vi "Base Set Run Java Script Error.vi"(4 "error in":errorcluster, 5 "output file in":path, 6 "data in":T1, 7 "ATS Framework Fields in":T2) -> (0 "error out":errorcluster)   [LabVIEW 2019]
uses:
  ATS Framework Fields.ctl
  Run Tool Output.ctl
  <vilib>/regexp/Match Regular Expression.xnode
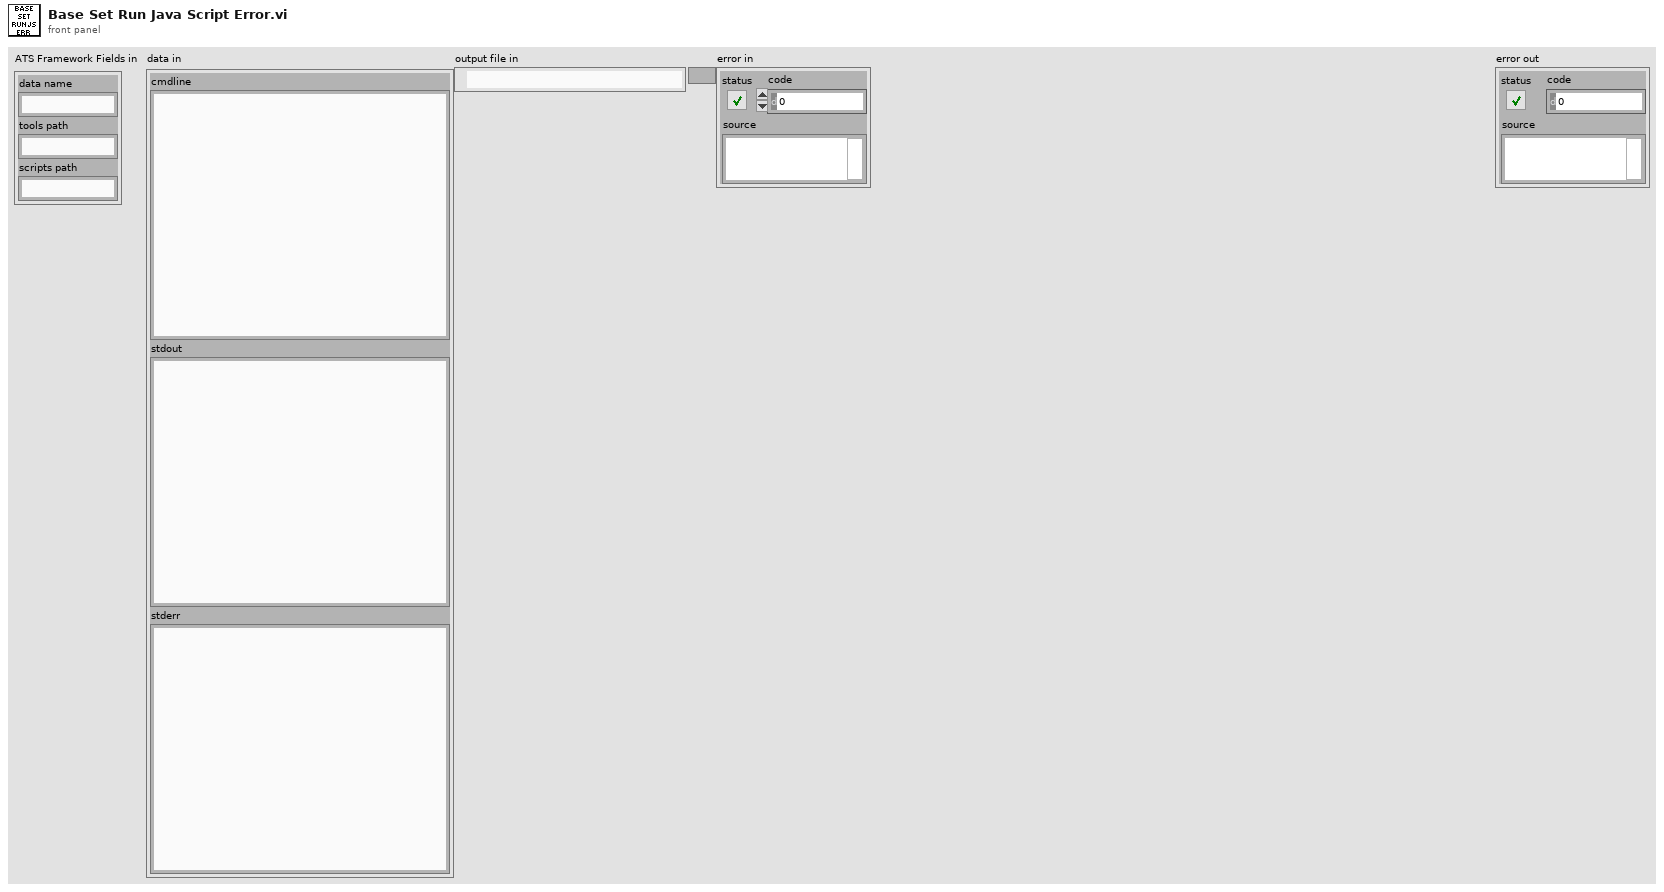
[diagram p1: front panel]
types:
  T1 = typedef "Run Tool Output.ctl" = cluster{"cmdline":string, "stdout":string, "stderr":string}
  T2 = typedef "ATS Framework Fields.ctl" = cluster{"data name":string, "tools path":string, "scripts path":string}
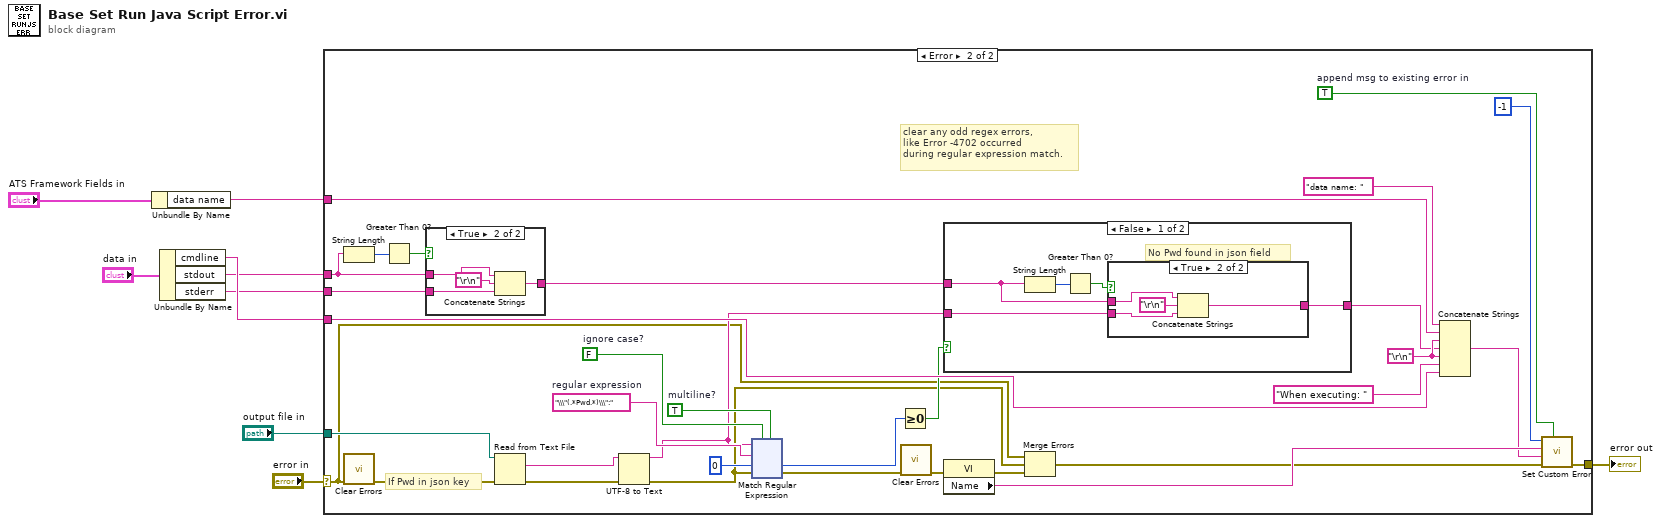
[diagram p0: block diagram]
diagram:
  n1 = Unbundle By Name("ATS Framework Fields in") -> ("data name"=w7:string)
  n2 = Unbundle By Name("data in") -> ("cmdline"=w5:string, "stdout"=w4:string, "stderr"=w3:string)
  n3 = case shown="Error" "error in" {
    selector: "error in" -> [w10 w17]
    tunnel: [w10 w36] -> w9
    tunnel: w7 -> [_ w43]
    tunnel: w4 -> [_ w13]
    tunnel: w5 -> [_ w32]
    tunnel: w3 -> [_ w12]
    tunnel: "output file in" -> [_ w19]
    frame No Error {
    }
    frame Error {
      w30 = "\\\"(.*Pwd.*)\\\":"  # regular expression
      w27 = FALSE  # ignore case?
      w28 = TRUE  # multiline?
      w35 = TRUE  # append msg to existing error in
      w41 = "\r\n"
      # "clear any odd regex errors,\nlike Error -4702 occurred\nduring regular expression match."
      # "If Pwd in json key"
      n4 = String Length(string=w13) -> (length=w15:i32)
      n5 = call <vilib>:"Clear Errors.vi"("error in (no error)"=w17) -> ("error out"=w20:errorcluster)  [unwired: 5 in, 1 out]
      n6 = Greater Than 0?(x=w15) -> (x > 0?=w14:bool)
      n7 = case shown="True" w14 {
        tunnel: w13 -> [_ w47]
        tunnel: [w44 w46] -> w11
        tunnel: w12 -> [w44 w45]
        frame False {
        }
        frame True {
          n8 = Concatenate Strings(w47, "\r\n", w45) -> (w46:string)
        }
      }
      n9 = Read from Text File(file (use dialog)=w19, error in=w20) -> (text=w21:string, error out=w22:errorcluster)  [unwired: 2 in, 2 out]
      n10 = UTF-8 to Text(8:w22, 11:w21) -> (0:w16:errorcluster, 3:w18:string)  [unwired: 1 in]
      n11 = xnode "Match Regular Expression"("input string"=w18, "regular expression"=w30, "offset (0)"=0 ("offset past match"), "error in"=w16, "ignore case? (F)"=w27, "multiline? (F)"=w28) -> ("offset past match"=w26:i32, "error out"=w25:errorcluster)  [unwired: 3 out]
      n12 = Greater Or Equal To 0?(x=w26) -> (x >= 0?=w24:bool)
      n13 = call <vilib>:"Clear Errors.vi"("error in (no error)"=w25) -> ("error out"=w23:errorcluster)  [unwired: 5 in, 1 out]
      n14 = case shown="False" w24 {
        tunnel: w18 -> [w164 _]
        tunnel: [w165 w173] -> w31
        tunnel: w11 -> [w163 w173]
        frame False {
          # "No Pwd found in json field"
          n15 = String Length(string=w163) -> (length=w167:i32)
          n16 = Greater Than 0?(x=w167) -> (x > 0?=w166:bool)
          n17 = case shown="True" w166 {
            tunnel: w163 -> [_ w171]
            tunnel: [w168 w170] -> w165
            tunnel: w164 -> [w168 w169]
            frame False {
            }
            frame True {
              n18 = Concatenate Strings(w171, "\r\n", w169) -> (w170:string)
            }
          }
        }
        frame True {
          # "Pwd found in json field.\nThis vi does not hide Pwds,\nso we can't include the data\nin the error message here."
        }
      }
      n19 = property class="VI"(error in=w23) -> (error out=w40:errorcluster, "Name"=w39:string)  [unwired: 1 in, 1 out]
      n20 = Merge Errors(w17, w16, w40) -> (w34:errorcluster)
      n21 = Concatenate Strings("data name: " ("string"), w43, w41, w31, w41, "When executing: " ("string"), w32) -> (w37:string)
      n22 = call "Set Custom Error.vi"("append msg to existing error in"=w35, "error in"=w34, "message in"=w37, "source in"=w39, "code in"=-1 ("code")) -> ("error out"=w36:errorcluster)  [unwired: 6 in]
    }
  }
  "error out" <- w9
